vi "SAP.vi"(8 "error in (no error)":errorcluster, 11 "input":T2) -> (0 "error out":errorcluster, 3 "output":T1)   [LabVIEW 2023]
uses:
  <userlib>/WebService/_SAP/SAP.lvlib
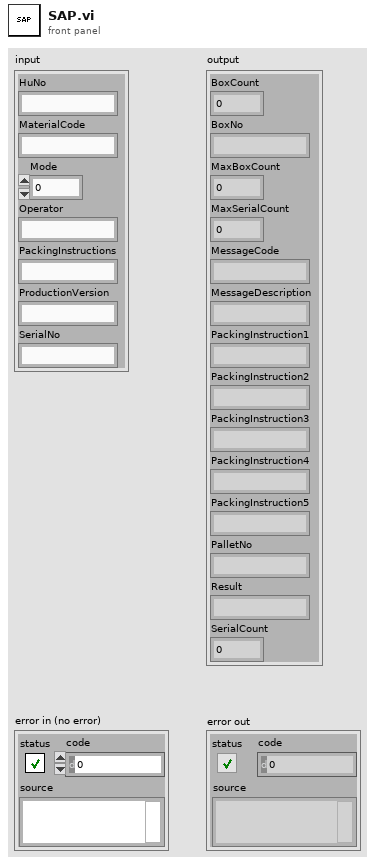
[diagram p1: front panel]
types:
  T1 = cluster{"BoxCount":i32, "BoxNo":string, "MaxBoxCount":i32, "MaxSerialCount":i32, "MessageCode":string, "MessageDescription":string, "PackingInstruction1":string, "PackingInstruction2":string, "PackingInstruction3":string, "PackingInstruction4":string, "PackingInstruction5":string, "PalletNo":string, "Result":string, "SerialCount":i32}
  T2 = cluster{"HuNo":string, "MaterialCode":string, "Mode":i32, "Operator":string, "PackingInstructions":string, "ProductionVersion":string, "SerialNo":string}
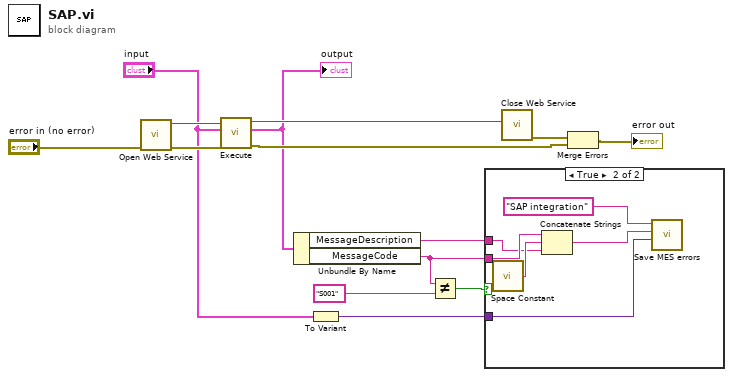
[diagram p0: block diagram]
diagram:
  n1 = call <userlib>:"Open Web Service.vi"("error in (no error)"="error in (no error)") -> ("error out"=w13:errorcluster, "SAP refnum"=w14:refnum<k24>)  [unwired: 9 in]
  n2 = call <userlib>:"Execute.vi"("error in (no error)"=w13, ".NET:ContactAndRegisterWithNmaSapService.SerialNoRegisterRequest"="input", "SAP refnum"=w14) -> ("error out"=w10:errorcluster, ".NET:ContactAndRegisterWithNmaSapService.SerialNoRegisterResponse"=w6:T1, "SAP refnum out"=w12:refnum<k24>)  [unwired: 6 in]
  "output" <- w6
  n3 = Unbundle By Name(w6) -> ("MessageDescription"=w4:string, "MessageCode"=w3:string)
  n4 = To Variant(anything="input") -> (Variant=w1:variant)
  n5 = Not Equal?(x=w3, y="S001") -> (x != y?=w7:bool)
  n6 = case shown="True" w7 {
    tunnel: w4 -> [_ w18]
    tunnel: w3 -> [_ w20]
    tunnel: w1 -> [_ w15]
    frame False {
    }
    frame True {
      n7 = call <vilib>:"Space Constant.vi"() -> ("String"=w19:string)
      n8 = Concatenate Strings(w20, w19, w18) -> (w17:string)
      n9 = call "Save MES errors.vi"("Sent parameters"=w15, "Error Text"=w17, "Operation"="SAP integration") -> ()  [unwired: 9 in]
    }
  }
  n10 = call <userlib>:"Close Web Service.vi"("SAP refnum"=w12) -> ("error out"=w11:errorcluster)  [unwired: 10 in]
  n11 = Merge Errors(w11, w10) -> (→"error out":errorcluster)
